vi "Method.vi"(4 "Value":refnum<class "Abs_Numeric.lvclass">) -> (1 "Result":refnum<class "ConvertTo_CPLX_DBL.lvclass">)   [LabVIEW 2021, in "ConvertTo_CPLX_DBL.lvclass"]
uses:
  ConvertTo_CPLX_DBL.lvclass
  Abs_Types/Numeric/Abs_Numeric.lvclass
  ConvertTo_CPLX_DBL.lvclass/ConvertTo_CPLX_DBL.ctl
  Properties/Write Value.vi
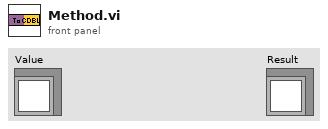
[diagram p1: front panel]
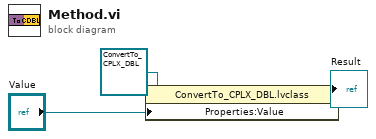
[diagram p0: block diagram]
diagram:
  n1 = property class="ConvertTo_CPLX_DBL.lvclass"(reference=refnum<class "ConvertTo_CPLX_DBL.lvclass"> refnum ("ConvertTo_DBL.lvclass"), "Properties:Value"="Value") -> (reference out=→"Result":refnum<class "ConvertTo_CPLX_DBL.lvclass">)  [unwired: 1 in, 1 out]
